vi "Read AOI list.vi"() -> (0 "Number of AOIs":i32)   [LabVIEW 2016]
doc: "Read AOI coordinates from a user-specified file and stores them in the global AOI list. Any existing AOIs are deleted. The first line of the external file is for the number of AOIs, but this is ignored and the number is obtained by counting lines. Each subsequent line has coordinates of an AOI (x, y, dx, dy). Note that the internal AOI list is stored in x1, y1, x2, y2 format."
uses:
  <vilib>/Utility/file.llb/Read From Spreadsheet File (DBL).vi
  AOI List Globals.vi
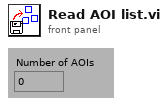
[diagram p1: front panel]
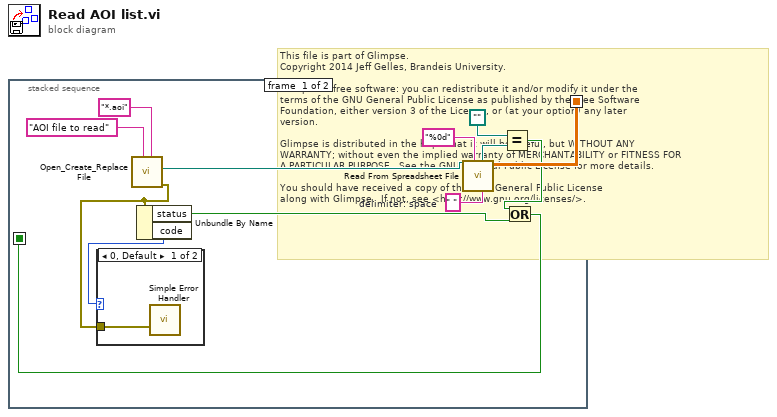
[diagram p0: block diagram]
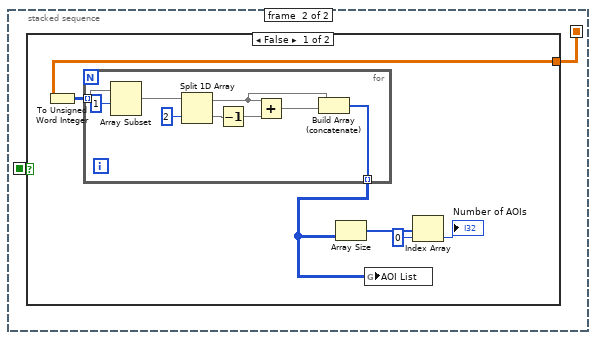
[diagram p3: hidden frame]
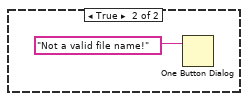
[diagram p4: hidden frame]
diagram:
  # "This file is part of Glimpse. \nCopyright 2014 Jeff Gelles, Brandeis University.    \n\nGlimpse is free software: you can redistribute it and/or modify it under the \nterms of the GNU General Public License as published by the Free Software \nFoundation, either version 3 of the License, or (at your option) any later \nversion.\n\nGlimpse is distributed in the hope that it will be useful, but WITHOUT ANY \nWARRANTY; without even the implied warranty of MERCHANTABILITY or FITNESS FOR \nA PARTICULAR PURPOSE.  See the GNU General Public License for more details.\n\nYou should have received a copy of the GNU General Public License\nalong with Glimpse.  If not, see <http://www.gnu.org/licenses/>."
  n1 = stacked-sequence {
    seq-local: [w10 _] -> [_ w16]
    seq-local: [w1 _] -> [_ w15]
    frame #0 {
      w13 = " "  # delimiter: space
      n2 = call <vilib>:"Open_Create_Replace File.vi"("pattern"="*.aoi", "prompt"="AOI file to read") -> ("error out"=w4:errorcluster, "new file path"=w8:path)  [unwired: 5 in, 3 out]
      n3 = Unbundle By Name(w4) -> ("status"=w3:bool, "code"=w5:i32)
      n4 = case shown="0, Default" w5 {
        tunnel: w4 -> [w14 _]
        frame 0, Default {
          n5 = call <vilib>:"Simple Error Handler.vi"("error in (no error)"=w14) -> ()  [unwired: 1 in, 8 out]
        }
        frame 43 {
        }
      }
      n6 = call-poly <vilib>:"Read From Spreadsheet File.vi"("delimiter (\\t)"=w13, "format (%.3f)"="%0d", "file path (dialog if empty)"=w8) -> ("all rows"=w10:dbl[][], "new file path (Not A Path if cancelled)"=w12:path)  [unwired: 2 in, 5 out]
      n7 = Equal?(x=path "", y=w12) -> (x = y?=w2:bool)
      n8 = Or(x=w2, y=w3) -> (x .or. y?=w1:bool)
    }
    frame #1 {
      n9 = case shown="False" w15 {
        tunnel: w16 -> [w17 _]
        frame False {
          n10 = To Unsigned Word Integer(number=w17) -> (unsigned 16bit integer=w22:u16[][])
          n11 = for {
            tunnel: w22 -> [w24] mode=indexing
            tunnel: [w26] -> w19 mode=indexing
            n12 = Array Subset(array=w24, index=1) -> (w25:u16[])  [unwired: 1 in]
            n13 = Split 1D Array(array=w25, index=2) -> (first subarray=w28:u16[], second subarray=w30:u16[])
            n14 = Decrement(x=w30) -> (x-1=w29:u16[])
            n15 = Add(x=w28, y=w29) -> (x+y=w27:u16[])
            n16 = Build Array (concatenate)(w28, w27) -> (w26:u16[])
          }
          n17 = Array Size(array=w19) -> (size(s)=w21:i32[])
          n18 = global write "AOI List Globals.vi" "AOI List"(w19) -> ()
          n19 = Index Array(array=w21, index=0) -> (element=→"Number of AOIs":i32)
        }
        frame True {
          n20 = One Button Dialog(message="Not a valid file name!") -> ()  [unwired: 2 out]
        }
      }
    }
  }
